vi "Queue References FGV.vi"(8 "error in":errorcluster, 11 "function":enum16{"obtain", "get", "release"}(ring)) -> (0 "error out":errorcluster, 3 "module queues":T1)   [LabVIEW 2017, in "WinHost.lvlib"]
uses:
  WinHost.lvlib
  Private TypeDefs/Module Queues.ctl
  Private TypeDefs/Message Queue Element.ctl
  Global TypeDefs/Registered Modules.ctl
  Public TypeDefs/Messages.ctl
  Private TypeDefs/STM Queue Element.ctl
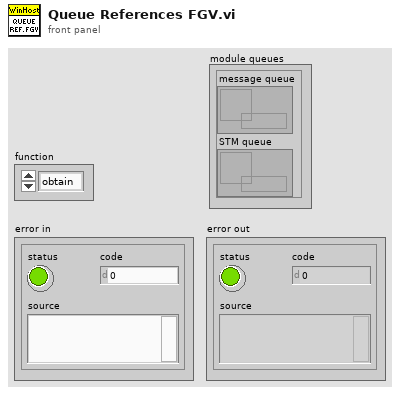
[diagram p1: front panel]
types:
  T1 = typedef "WinHost.lvlib/Module Queues.ctl" = cluster{"message queue":refnum<queue>, "STM queue":refnum<queue>}
  T2 = typedef "WinHost.lvlib/STM Queue Element.ctl" = cluster{"name":string, "data":string, "stop":bool}
  T3 = typedef "WinHost.lvlib/Message Queue Element.ctl" = cluster{"source":T4, "message":T5, "data":variant}
  T4 = typedef "Registered Modules.ctl" = enum16{"Controller", "DAQ", "Error Handler", "Game", "myPAM", "WinHost", "Logger"}
  T5 = typedef "WinHost.lvlib/Messages.ctl" = enum16{"shutdown", "wait for host", "communicate"}
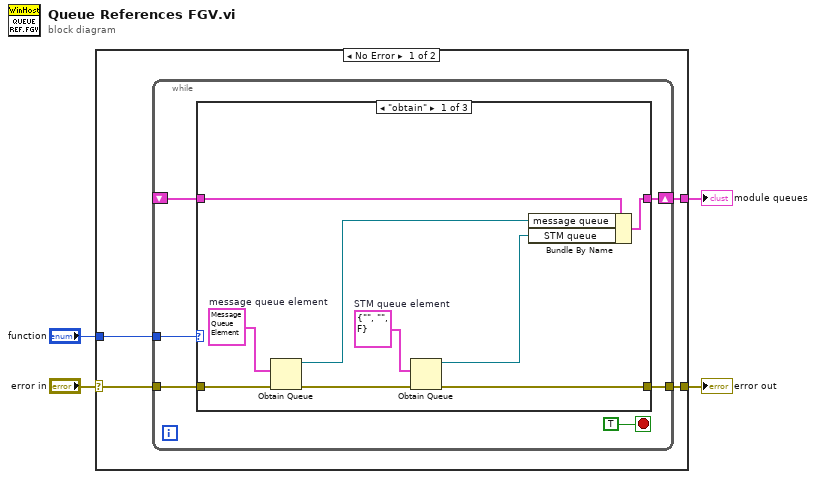
[diagram p0: block diagram]
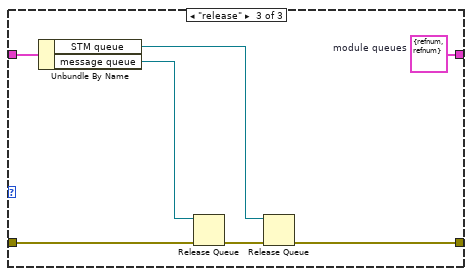
[diagram p3: hidden frame]
diagram:
  n1 = case shown="No Error" "error in" {
    selector: "error in" -> [w8 w33]
    tunnel: [w7 w33] -> w3
    tunnel: "function" -> [w6 _]
    tunnel: [w5 _] -> w1
    frame No Error {
      n2 = while {
        tunnel: w8 -> [w13]
        tunnel: [w12] -> w7
        tunnel: w6 -> [w11]
        shift-right: [w10] -> w5
        shift-left: _ -> [w9]
        stop <- TRUE stop-if-true
        n3 = case shown="\"obtain\"" w11 {
          tunnel: w13 -> [w23 w25 w32]
          tunnel: [w15 w25 w27] -> w12
          tunnel: [w19 w24 w29] -> w10
          tunnel: w9 -> [w21 w24 w31]
          frame "obtain" {
            w18 = T2 {"name"="", "data"="", "stop"=FALSE}  # STM queue element
            w22 = T3 {"source"=enum."Controller", "message"=enum."shutdown", "data"=variant}  # message queue element
            n4 = Obtain Queue(element data type=w22, error in (no error)=w23) -> (queue out=w20:refnum<queue>, error out=w17:errorcluster)  [unwired: 3 in, 1 out]
            n5 = Obtain Queue(element data type=w18, error in (no error)=w17) -> (queue out=w16:refnum<queue>, error out=w15:errorcluster)  [unwired: 3 in, 1 out]
            n6 = Bundle By Name(cluster=w21, "message queue"=w20, "STM queue"=w16) -> (w19:T1)
          }
          frame "get", Default {
          }
          frame "release" {
            w29 = T1 {"message queue"=refnum, "STM queue"=refnum}  # module queues
            n7 = Unbundle By Name(w31) -> ("STM queue"=w26:refnum<queue>, "message queue"=w30:refnum<queue>)
            n8 = Release Queue(queue=w30, error in (no error)=w32) -> (error out=w28:errorcluster)  [unwired: 1 in, 2 out]
            n9 = Release Queue(queue=w26, error in (no error)=w28) -> (error out=w27:errorcluster)  [unwired: 1 in, 2 out]
          }
        }
      }
    }
    frame Error {
    }
  }
  "error out" <- w3
  "module queues" <- w1
